vi "copy.vi"(8 "error in (no error)":errorcluster, 10 "ScriptEventForCopy":refnum<class "ScriptEvent.lvclass">, 11 "Delay in":refnum<class "Delay.lvclass">) -> (0 "error out":errorcluster, 3 "Delay Copy":refnum<class "Delay.lvclass">)   [LabVIEW 2011, in "Tools.lvlib" / "Scripting.lvlib" / "Delay.lvclass"]
uses:
  Delay.lvclass
  ScriptEvent.lvclass
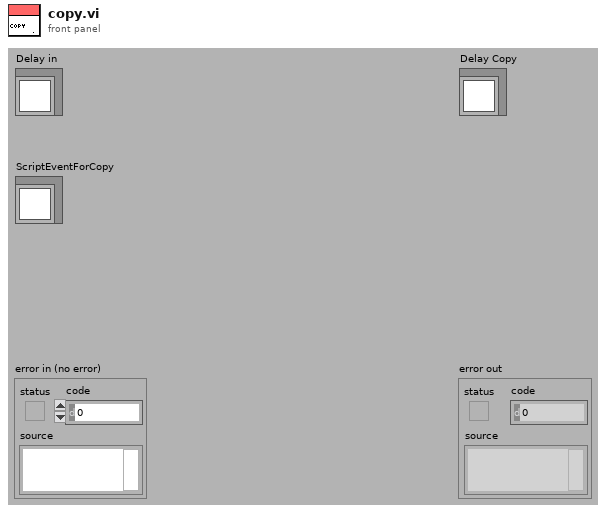
[diagram p1: front panel]
types:
  T1 = enum16{"changeValue", "pulse", "clock", "rampUp", "rampDown", "singleTone", "singleToneRamp", "playFile", "rf", "rfRamp", "delay"}
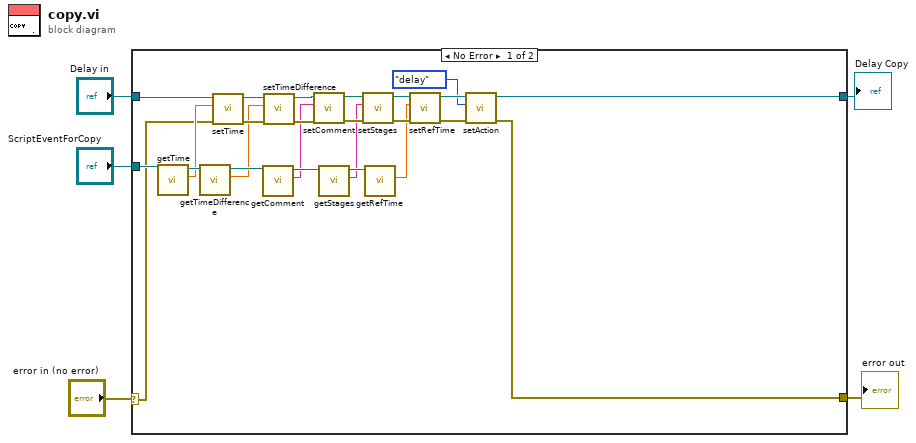
[diagram p0: block diagram]
diagram:
  n1 = case shown="No Error" "error in (no error)" {
    selector: "error in (no error)" -> [w11 w32]
    tunnel: [w9 w31] -> w5
    tunnel: "Delay in" -> [w25 w31]
    tunnel: [w8 w32] -> w2
    tunnel: "ScriptEventForCopy" -> [w30 _]
    frame No Error {
      n2 = call "getTime.vi"("ScriptEvent.lvclass in"=w30) -> ("time"=w24:dbl, "ScriptEvent.lvclass out"=w29:refnum<class "ScriptEvent.lvclass">)  [unwired: 8 in, 1 out]
      n3 = call "getTimeDifference.vi"("ScriptEvent.lvclass in"=w29) -> ("time difference"=w21:dbl, "ScriptEvent.lvclass out"=w28:refnum<class "ScriptEvent.lvclass">)  [unwired: 8 in, 1 out]
      n4 = call "setTime.vi"("error in (no error)"=w11, "time"=w24, "ScriptEvent.lvclass in"=w25) -> ("error out"=w22:errorcluster, "ScriptEvent.lvclass out"=w23:refnum<class "Delay.lvclass">)  [unwired: 7 in]
      n5 = call "getComment.vi"("ScriptEvent.lvclass in"=w28) -> ("comment"=w18:string, "ScriptEvent.lvclass out"=w27:refnum<class "ScriptEvent.lvclass">)  [unwired: 8 in, 1 out]
      n6 = call "setTimeDifference.vi"("error in (no error)"=w22, "time difference"=w21, "ScriptEvent.lvclass in"=w23) -> ("error out"=w19:errorcluster, "ScriptEvent.lvclass out"=w20:refnum<class "Delay.lvclass">)  [unwired: 7 in]
      n7 = call-dynamic "setComment.vi"("error in (no error)"=w19, "comment"=w18, "ScriptEvent.lvclass in"=w20) -> ("error out"=w16:errorcluster, "ScriptEvent.lvclass out"=w17:refnum<class "Delay.lvclass">)  [unwired: 7 in]
      n8 = call "getStages.vi"("ScriptEvent.lvclass in"=w27) -> ("Stage"=w15:string, "ScriptEvent.lvclass out"=w26:refnum<class "ScriptEvent.lvclass">)  [unwired: 8 in, 1 out]
      n9 = call-dynamic "setStages.vi"("error in (no error)"=w16, "Stage"=w15, "ScriptEvent.lvclass in"=w17) -> ("error out"=w13:errorcluster, "ScriptEvent.lvclass out"=w14:refnum<class "Delay.lvclass">)  [unwired: 7 in]
      n10 = call "getRefTime.vi"("ScriptEvent.lvclass in"=w26) -> ("refTime"=w12:dbl)  [unwired: 8 in, 2 out]
      n11 = call "setRefTime.vi"("error in (no error)"=w13, "refTime"=w12, "ScriptEvent.lvclass in"=w14) -> ("error out"=w7:errorcluster, "ScriptEvent.lvclass out"=w10:refnum<class "Delay.lvclass">)  [unwired: 7 in]
      n12 = call "setAction.vi"("error in (no error)"=w7, "action"=T1."delay", "ScriptEvent.lvclass in"=w10) -> ("error out"=w8:errorcluster, "ScriptEvent.lvclass out"=w9:refnum<class "Delay.lvclass">)  [unwired: 7 in]
    }
    frame Error {
    }
  }
  "error out" <- w2
  "Delay Copy" <- w5
